vi "GetTimeSubVI.vi"() -> (3 "Seconds":dbl)   [LabVIEW 2019, in "Chapter2-Ex1-Library.lvlib"]
uses:
  Chapter2-Ex1-Library.lvlib
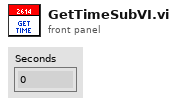
[diagram p1: front panel]
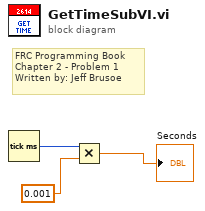
[diagram p0: block diagram]
diagram:
  # "FRC Programming Book\nChapter 2 - Problem 1\nWritten by: Jeff Brusoe"
  n1 = Tick Count (ms)() -> (millisecond timer value=w1:u32)
  n2 = Multiply(x=w1, y=0.001) -> (x*y=→"Seconds":dbl)
